vi "Verify Measurement Logic.vi"(6 "averaging parameters":T2, 7 "Measure Call Context in":refnum<class "Measure Call Context.lvclass">, 8 "error in":errorcluster, 9 "window and overlap":cluster{"window":u32, "overlap":dbl}, 11 "DAQmx Configuration":T4 {"Run Mode" items=["Run Once", "Continuously"]; "Block Size" min=0; "Sample Rate (Hz)" min=0.0; "Trigger Type" items=["None", "Analog Reference"]; "Channel Table"."input terminal configuration" items=["default"=-1, "RSE"=10083, "NRSE"=10078, "Differential"=10106, "Pseudodifferential"=12529]; "Channel Table"."Channel Type" items=["Voltage (V)"=0, "Charge (C)"=9, "-"=99, "SPL (Pa)"=3, "Force (lbf)"=6, "Force (N)"=1, "Acceleration (g) - IEPE"=2, "Acceleration (g) - Charge"=12, "Acceleration (g) - 4 wire DC Voltage"=22, "Velocity (in/s)"=7, "Velocity (mm/s)"=8, "Prox Probe (mil)"=4, "Prox Probe (mm)"=5]}) -> (0 "error out":errorcluster, 3 "last measurement results":T1, 4 "stop channel":T3)   [LabVIEW 2024, in "Dynamic Signal Acquisition (Interactive).lvlib"]
uses:
  Dynamic Signal Acquisition (Interactive).lvlib
  Dynamic Signal Acquisition (Interactive) UI/SFPDAQ Configuration.ctl
  Dynamic Signal Acquisition (Interactive) UI/SFPDAQmx Channel Info.ctl
  <extravilib>/ChannelInstances/Tag-bool/))Channel.ctl
  <vilib>/Plug-In SDKs/Measurements/Measure Call Context/Measure Call Context.lvclass
  Measurement Results.ctl
  <extravilib>/ChannelInstances/Messenger-a[.](wfm(dbl))/Instantiate.vi
  DSA_CFG_ACQ.lvlib
  Dynamic Signal Acquisition (Interactive) UI/Dynamic Signal Acquisition (Interactive) UI.lvlib
  <extravilib>/ChannelInstances/Tag-bool.lvlib
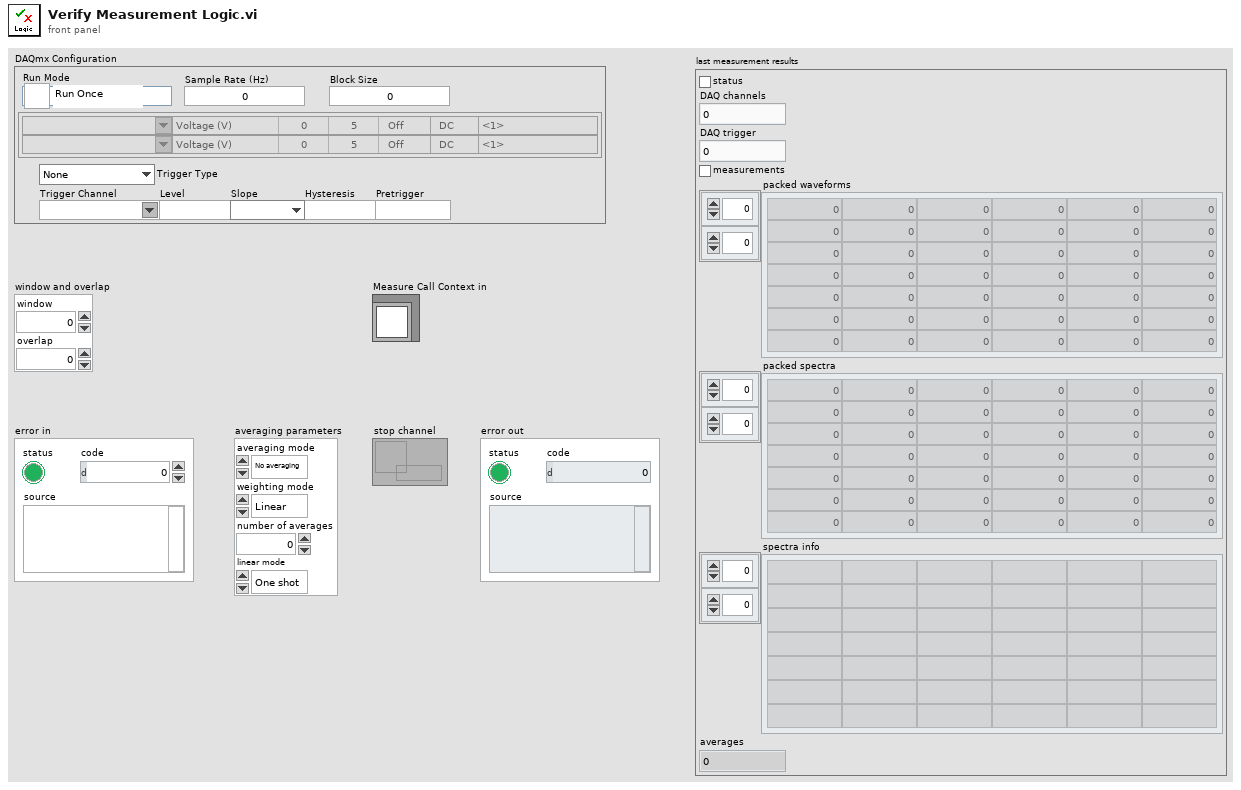
[diagram p1: front panel]
types:
  T1 = typedef "Dynamic Signal Acquisition (Interactive).lvlib/Measurement Results.ctl" = cluster{"status":bool, "DAQ channels":u32, "DAQ trigger":u32, "measurements":bool, "packed waveforms":dbl[][], "packed spectra":dbl[][], "spectra info":string[][], "averages":dbl}
  T2 = cluster{"averaging mode":enum16{"No averaging", "Vector averaging", "RMS averaging", "Peak hold"}, "weighting mode":enum16{"Linear", "Exponential"}, "number of averages":u32, "linear mode":enum16{"One shot", "Auto restart"}}
  T3 = typedef "Tag-bool.lvlib/))Channel.ctl" = refnum<queue>
  T4 = typedef "Dynamic Signal Acquisition (Interactive) UI.lvlib/SFPDAQ Configuration.ctl" = cluster{"Run Mode":u16, "Sample Rate (Hz)":dbl, "Block Size":i32, "Channel Table":T5[], "Trigger Type":u16, "Trigger Channel":string, "Level":dbl, "Pretrigger":i32, "Hysteresis":dbl, "Slope":enum16{"Falling", "Rising"}}
  T5 = typedef "Dynamic Signal Acquisition (Interactive) UI.lvlib/SFPDAQmx Channel Info.ctl" = cluster{"DAQmx Channel":tag, "Channel Type":u16, "Max":dbl, "Sensitivity":dbl, "Coupling":enum16{"AC", "DC"}, "input terminal configuration":i32, "excitation":enum16{"Off", "Min", "Max"}}
  T6 = typedef "Messenger-a[.](wfm(dbl)).lvlib/))Channel.ctl" = refnum<queue>
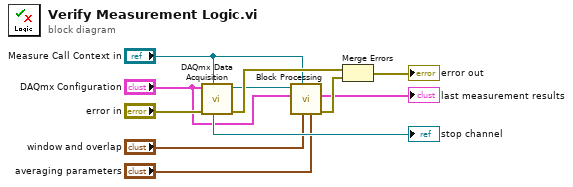
[diagram p0: block diagram]
diagram:
  n1 = call "DAQmx Data Acquisition.vi"("measure call context in"="Measure Call Context in", "error in"="error in", "DAQmx Cfg"="DAQmx Configuration") -> ("error out"=w7:errorcluster, "waveforms channel"=w6:T6, "stop channel"=→"stop channel":T3)  [unwired: 6 in]
  n2 = call "Block Processing.vi"("averaging parameters"="averaging parameters", "window and overlap"="window and overlap", "measure call context"="Measure Call Context in", "DAQmx Configuration"="DAQmx Configuration", "data to process"=w6) -> ("error out"=w8:errorcluster, "last measurement results"=→"last measurement results":T1)  [unwired: 5 in]
  n3 = Merge Errors(w7, w8) -> (→"error out":errorcluster)
